vi "Actuator To Cylinder.vi"(8 "error in (no error)":errorcluster, 9 "Lateral Force":dbl[unit] format="%.3f", 10 "Axial Force":dbl[unit] format="%.3f", 11 "Actuator To Cylinder Forces in":refnum<class "Actuator To Cylinder Forces.lvclass">) -> (0 "error out":errorcluster, 1 "FC2 Value":dbl format="%.3f", 2 "FC1 Value":dbl format="%.3f", 3 "Actuator To Cylinder Forces out":refnum<class "Actuator To Cylinder Forces.lvclass">)   [LabVIEW 2015, in "Actuator To Cylinder Forces.lvclass"]
uses:
  Actuator To Cylinder Forces.lvclass
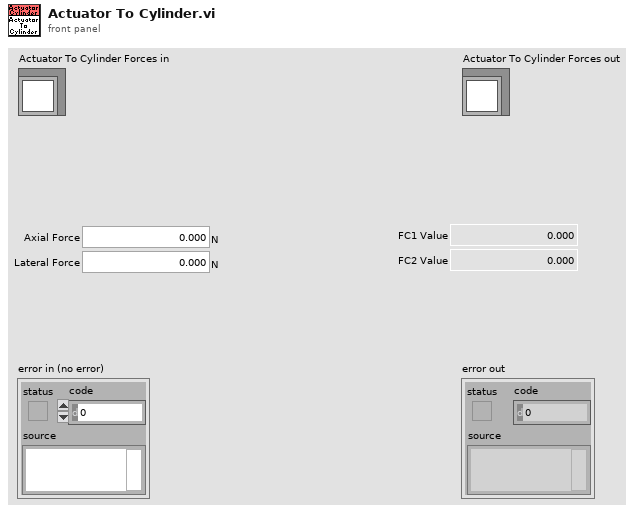
[diagram p1: front panel]
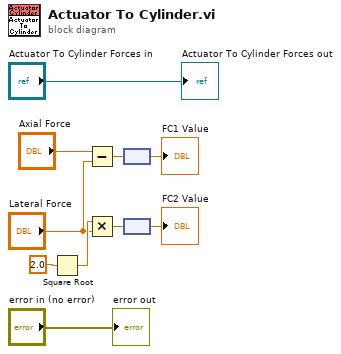
[diagram p0: block diagram]
diagram:
  n1 = Square Root(x=2.0) -> (sqrt(x)=w6:dbl)
  n2 = Subtract(x="Axial Force", y="Lateral Force") -> (x-y=w4:dbl[unit])
  n3 = Multiply(x=w6, y="Lateral Force") -> (x*y=w2:dbl[unit])
  n4 = node(w4) -> (→"FC1 Value":dbl)
  n5 = node(w2) -> (→"FC2 Value":dbl)
  "error out" <- "error in (no error)"
  "Actuator To Cylinder Forces out" <- "Actuator To Cylinder Forces in"
